vi "Begin.vi"(8 "error in":errorcluster) -> (0 "error out":errorcluster)   [LabVIEW 2016]
doc: "Called before other user functions, this VI is expected to open initial I/O refnums, load in file data, and do all program initialization. Notice that the <B>error out</B> terminal is simply used for data flow. Wiring it to other structures or subVIs ensures that this VI runs first."
uses:
  Refname/Queues.ctl
  Refname/Sensors.ctl
  Refname/Refname to String (Queues).vi
  Robot Global Data.vi
  Refname/Refname to String (Sensors).vi
  <vilib>/Rock Robotics/WPI/Joystick/WPI_JoystickDeviceEnum.ctl
  <vilib>/Rock Robotics/WPI/DriverStation/WPI_DriverStationRobotMode2.ctl
  <vilib>/Rock Robotics/WPI/ThirdParty/CanMotor/TalonSRX/WPI_CANTalonSRX_APIControlMode.ctl
  Refname/Motors.ctl
  <vilib>/Rock Robotics/WPI/SafetyOutput/WPI_SafetyOutputConfigMenu.ctl
  Refname/Controllers.ctl
  Refname/Refname to String (Motors).vi
  <vilib>/Rock Robotics/WPI/ThirdParty/CanMotor/TalonSRX/WPI_CANTalonSRX_APIFeedbackSelect.ctl
  <vilib>/Rock Robotics/WPI/ThirdParty/Sensors/ADIS16448 IMU/ADIS16448_IMU.lvlib
  <vilib>/Rock Robotics/SystemInterfaces/spilib/spi_bus.ctl
  Refname/Refname to String (Controllers).vi
panel:
  in  "Values to Log":string="TimeStamp, X, Y, Z, a, b, c, d, setpoint 1, setpoint 2, setpoint 3, setpoint 4, wheel power 1, wheel power 2, wheel power 3, wheel power 4, swerve current 1, swerve current 2, swerve current 3, swerve current 4"
  in  "PID gains":T1={"proportional gain (Kc)"=5.0, "integral time (Ti, min)"=0.032, "derivative time (Td, min)"=0.0} {"derivative time (Td, min)" format="%.3f"; "integral time (Ti, min)" format="%.8f"; "proportional gain (Kc)" format="%.8f"}
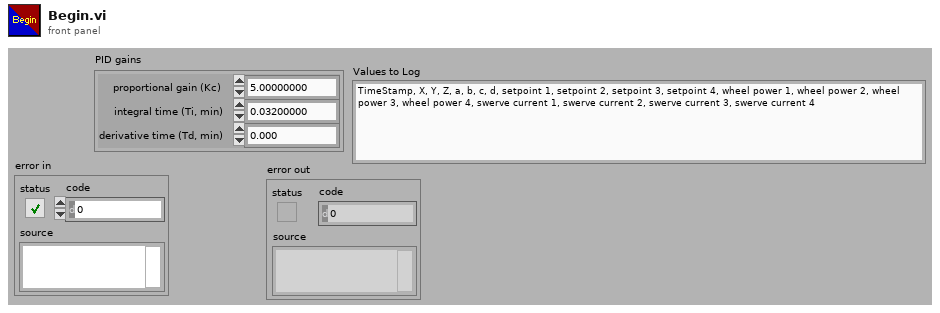
[diagram p1: front panel]
types:
  T1 = cluster{"proportional gain (Kc)":dbl, "integral time (Ti, min)":dbl, "derivative time (Td, min)":dbl}
  T2 = typedef "Queues.ctl" = enum16{"Log Queue"}
  T3 = cluster{"connection ID":refnum<k5>, "Running?":bool, "TCP Port":u16, "LastMessageReceivedTime":dbl, "WantsAppRestart":bool, "IsConnect":bool, "Vision Updates":cluster{"CapturedAgoMs":i32, "Valid?":bool, "CapturedAtTimestamp":dbl, "Targets":cluster{"X":dbl, "Y":dbl, "Z":dbl}[]}[]}
  T4 = typedef "WPI_SafetyOutputConfigMenu.ctl" = enum16{"Enable", "Disable"}
  T5 = typedef "Motors.ctl" = enum16{"Wheel 1", "Swerve 1", "Wheel 2", "Swerve 2", "Wheel 3", "Swerve 3", "Wheel 4", "Swerve 4", "Climber"}
  T6 = typedef "WPI_CANTalonSRX_APIControlMode.ctl" = enum8{"Percent VBus", "Speed", "Position", "Slave", "Unchanged / Invalid", "Voltage Compensation", "Current", "Motion Profile", "Motion Magic"}
  T7 = typedef "Sensors.ctl" = enum16{"DIP 1", "DIP 2", "DIP 3", "DIP 4", "IMU", "HuskieBoard"}
  T8 = typedef "spi_bus.ctl" = enum16{"SPI On-Board, CS0", "SPI On-Board, CS1", "SPI On-Board, CS2", "SPI On-Board, CS3", "SPI MXP", "Invalid"}
  T9 = typedef "WPI_DriverStationRobotMode2.ctl" = enum16{"Autonomous Disabled", "Autonomous Enabled", "Teleop Disabled", "Teleop Enabled", "Disconnected", "Finish", "Test Disabled", "Test Enabled", "Emergency Stopped"}
  T10 = typedef "WPI_CANTalonSRX_APIFeedbackSelect.ctl" = enum16{"Digital Quadrature Encoder", "Analog Potentiometer", "Analog Encoder", "Count on Quad-A (Rising-Edge)", "Count on Quad-A (Falling-Edge)", "CTR Magnetic Enc (Absolute)", "CTR Magnetic Enc (Relative)", "Pulse Width"}
  T11 = typedef "WPI_JoystickDeviceEnum.ctl" = enum16{"USB 0", "USB 1", "USB 2", "USB 3", "USB 4", "USB 5"}
  T12 = typedef "Controllers.ctl" = enum16{"Controller 0", "Controller 1"}
  T13 = typedef "WPI_MotorControlDeviceRef.ctl" = cluster{"DeviceStatus":errorcluster, "Type":T14, "PWM":cluster{"PWM Channel":T15, "DeadBand":T16}, "CAN":cluster{"Device Number":u8, "SetOutput VI Ref":variant, "GetOutput VI Ref":variant, "Enable VI Ref":variant, "Disable VI Ref":variant, "Data":variant}, "Invert":bool}
  T14 = typedef "WPI_MotorControlType.ctl" = enum16{"PWM", "CAN"}
  T15 = typedef "FPGA_DIOPWMChannel.ctl" = enum8{"PWM 0", "PWM 1", "PWM 2", "PWM 3", "PWM 4", "PWM 5", "PWM 6", "PWM 7", "PWM 8", "PWM 9", "PWM MXP 0", "PWM MXP 1", "PWM MXP 2", "PWM MXP 3", "PWM MXP 4", "PWM MXP 5", "PWM MXP 6", "PWM MXP 7", "PWM MXP 8", "PWM MXP 9", "Invalid"}
  T16 = typedef "WPI_PWMDeadband.ctl" = cluster{"Name":string, "maxPositivePwm":i32, "minPositivePwm":i32, "centerPwm":i32, "maxNegativePwm":i32, "minNegativePwm":i32, "angularRange":u16}
  T17 = typedef "WPI_JoystickDevRef.ctl" = cluster{"Device":T11}
  T18 = typedef "ADIS16448_IMU.lvlib/ADI_IMU_ADIS16448_InterruptDevRef.ctl" = cluster{"ADI IMU DevRef":T19, "InterruptRef":T20}
  T19 = typedef "ADIS16448_IMU.lvlib/ADI_IMU_ADIS16448_IMUDevRef.ctl" = cluster{"DevStatus":errorcluster, "Handle":i32, "SPI Bus":T8, "Device Found":bool, "Device Ready":bool, "Yaw Axis":enum16{"X", "Y", "Z"}, "AHRS Algorithm":enum16{"Complementary", "Madgwick"}, "Serial":u16, "Lot ID 2":u16, "Lot ID 1":u16, "Product ID":u16}
  T20 = typedef "WPI_InterruptRef.ctl" = cluster{"DevStatus":errorcluster, "InterruptIndex":T21}
  T21 = typedef "FPGA_InterruptIndex.ctl" = enum8{"0", "1", "2", "3", "4", "5", "6", "7", "Invalid"}
  T22 = typedef "WPI_SerialPortRef.ctl" = cluster{"DevStatus":errorcluster, "Serial Port Name":refnum<visa-resource-name>}
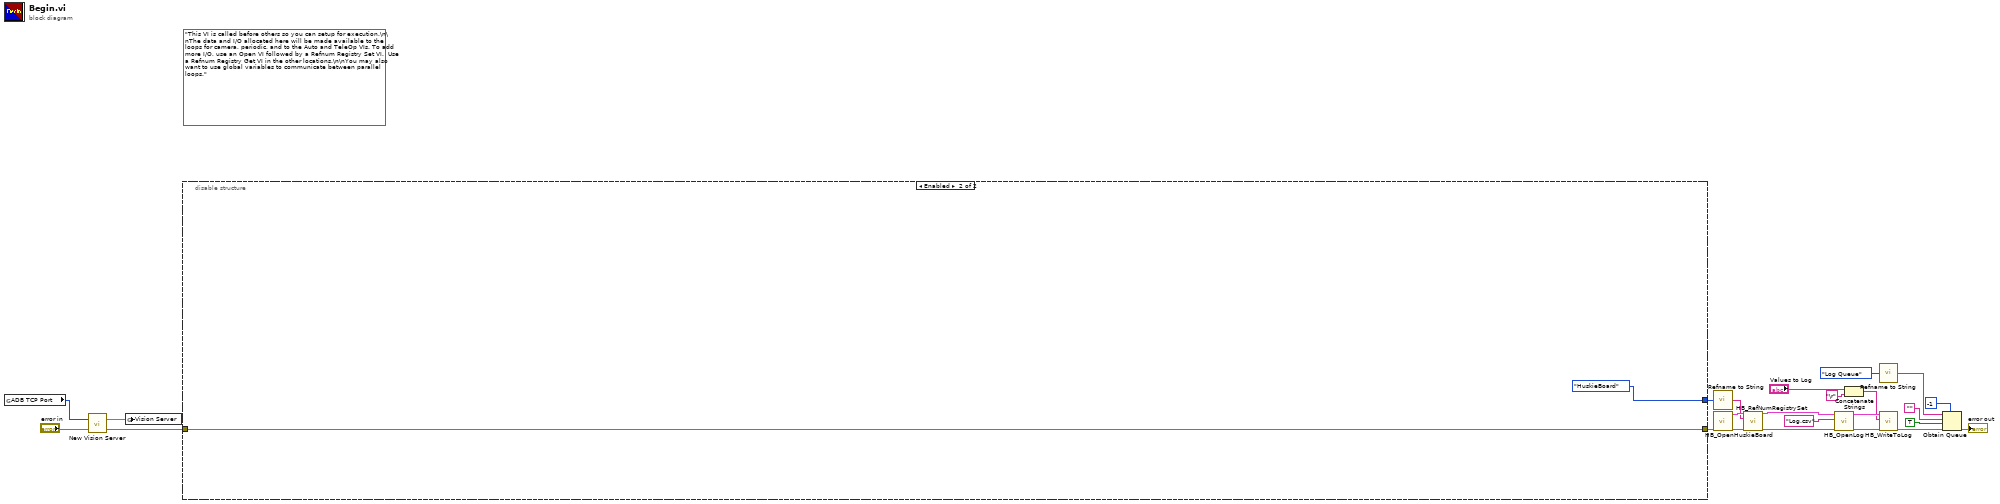
[diagram p0: block diagram]
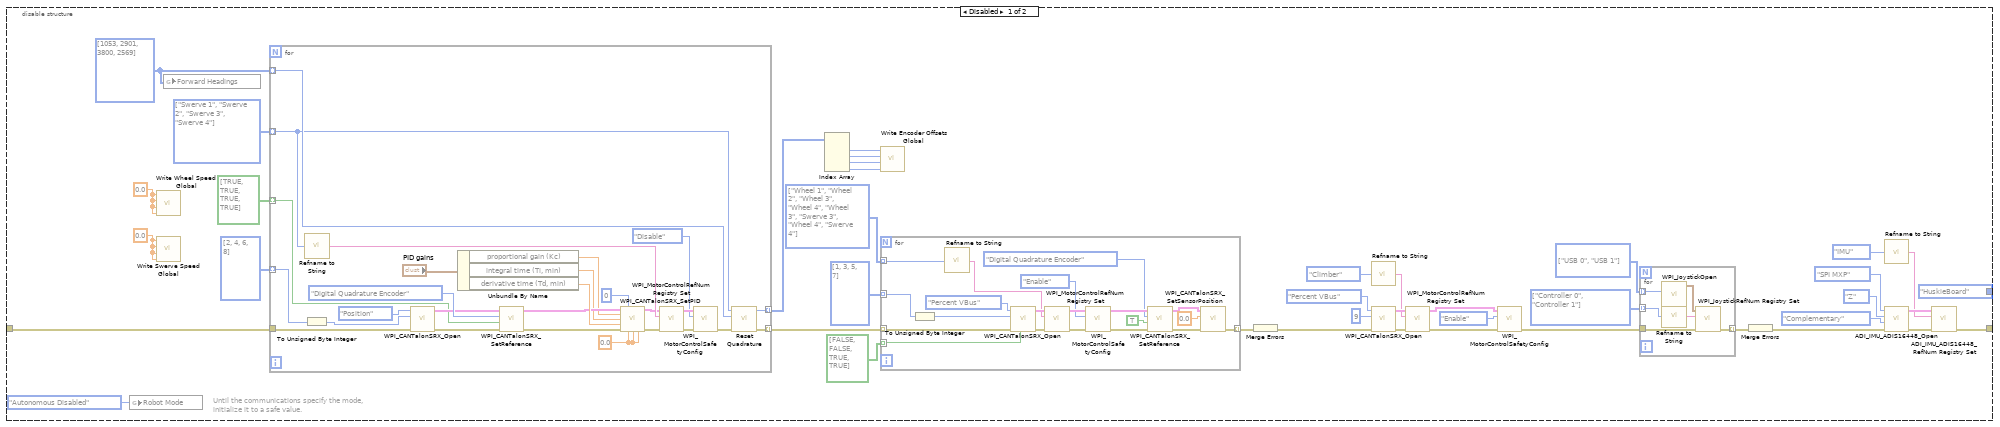
[diagram p2: hidden frame]
diagram:
  (unwired) "This VI is called before others so you can setup for execution.\n\nThe data and I/O allocated here will be made available to the loops for camera, periodic, and to the Auto and TeleOp VIs. To add more I/O, use an Open VI followed by a Refnum Registry Set VI.  Use a Refnum Registry Get VI in the other locations.\n\nYou may also want to use global variables to communicate between parallel loops."
  n1 = global read "Robot Global Data.vi" "ADB TCP Port"() -> (w11:u16)
  n2 = call "New Vision Server.vi"("error in"="error in", "TCP Port"=w11) -> ("error out"=w14:errorcluster, "Vision Server"=w13:T3)
  n3 = global write "Robot Global Data.vi" "Vision Server"(w13) -> ()
  n4 = disable-structure shown="Enabled" {
    disable-tunnel: [Sensors."HuskieBoard" ("Enum") Sensors."HuskieBoard" ("Enum")] -> w20
    disable-tunnel: w14 -> [w47 w121]
    disable-tunnel: [w46 w121] -> w10
    frame Disabled {
      w53 = i32[] [1053, 2901, 3800, 2569]
      w57 = 0.0
      w54 = 0.0
      w61 = T5[] [enum."Swerve 1", enum."Swerve 2", enum."Swerve 3", enum."Swerve 4"] items=["Wheel 1", "Swerve 1", "Wheel 2", "Swerve 2", "Wheel 3", "Swerve 3", "Wheel 4", "Swerve 4", "Climber"]
      w63 = T11[] [enum."USB 0", enum."USB 1"] items=["USB 0", "USB 1", "USB 2", "USB 3", "USB 4", "USB 5"]
      w64 = T12[] [enum."Controller 0", enum."Controller 1"] items=["Controller 0", "Controller 1"]
      w65 = T5[] [enum."Wheel 1", enum."Wheel 2", enum."Wheel 3", enum."Wheel 4", enum."Wheel 3", enum."Swerve 3", enum."Wheel 4", enum."Swerve 4"] items=["Wheel 1", "Swerve 1", "Wheel 2", "Swerve 2", "Wheel 3", "Swerve 3", "Wheel 4", "Swerve 4", "Climber"]
      # "Until the communications specify the mode,\ninitialize it to a safe value."
      n5 = global write "Robot Global Data.vi" "Robot Mode"(WPI_DriverStationRobotMode2."Autonomous Disabled" ("Robot Mode")) -> ()
      n6 = call "Write Wheel Speed Global.vi"("Wheel 4"=w54, "Wheel 3"=w54, "Wheel 2"=w54, "Wheel 1"=w54) -> ()
      n7 = call "Write Swerve Speed Global.vi"("Swerve 4"=w57, "Swerve 3"=w57, "Swerve 2"=w57, "Swerve 1"=w57) -> ()
      n8 = global write "Robot Global Data.vi" "Forward Headings"(w53) -> ()
      n9 = for {
        tunnel: w61 -> [w85] mode=indexing
        tunnel: i32[] [2, 4, 6, 8] -> [w88] mode=indexing
        tunnel: w47 -> [w87]
        tunnel: w53 -> [w86] mode=indexing
        tunnel: [w83] -> w55 mode=indexing
        tunnel: [w82] -> w58 mode=indexing
        tunnel: bool[] [TRUE, TRUE, TRUE, TRUE] -> [w77] mode=indexing
        w74 = 0.0 ("Output")
        n10 = To Unsigned Byte Integer(number=w88) -> (unsigned 8bit integer=w89:u8)
        n11 = call-poly "Refname to String.vi"("Enum"=w85) -> ("String"=w78:string)
        n12 = call <vilib>:"WPI_CANTalonSRX_Open.vi"("error in"=w87, "Device Number"=w89, "Control Mode"=WPI_CANTalonSRX_APIControlMode."Position") -> ("error out"=w79:errorcluster, "CAN Talon SRX Ref"=w80:T13)  [unwired: 7 in]
        n13 = Unbundle By Name("PID gains") -> ("proportional gain (Kc)"=w69:dbl, "integral time (Ti, min)"=w70:dbl, "derivative time (Td, min)"=w75:dbl)
        n14 = call <vilib>:"WPI_CANTalonSRX_SetReference.vi"("error in (no error)"=w79, "Reverse Feedback Sensor"=w77, "Feedback Reference"=WPI_CANTalonSRX_APIFeedbackSelect."Digital Quadrature Encoder", "CAN Talon SRX Ref"=w80) -> ("error out"=w72:errorcluster, "CAN Talon SRX Ref"=w73:T13)  [unwired: 6 in]
        n15 = call <vilib>:"WPI_CANTalonSRX_SetPID.vi"("CAN Talon SRX Ref"=w73, "Parameter Slot"=u8 0, "P"=w69, "I"=w70, "D"=w75, "error in (no error)"=w72, "F"=w74, "I Zone"=w74, "Ramp Rate"=w74) -> ("CAN Talon SRX Ref"=w67:T13, "error out"=w71:errorcluster)  [unwired: 5 in]
        n16 = call <vilib>:"WPI_MotorControlRefNum Registry Set.vi"("error in (no error)"=w71, "refnum name"=w78, "MotorControlDevRef"=w67) -> ("error out"=w92:errorcluster, "MotorControlDevRef"=w91:T13)  [unwired: 7 in]
        n17 = call <vilib>:"WPI_MotorControlSafetyConfig.vi"("error in (no error)"=w92, "mode"=WPI_SafetyOutputConfigMenu."Disable", "MotorControlDevRef"=w91) -> ("error out"=w84:errorcluster)  [unwired: 7 in, 1 out]
        n18 = call "Reset Quadrature.vi"("error in"=w84, "Forward Position"=w86, "Enum"=w85) -> ("error out"=w83:errorcluster, "Encoder Offset"=w82:i32)  [unwired: 7 in]
      }
      n19 = Index Array(array=w58) -> (element #1=w52:i32, element #2=w51:i32, element #3=w50:i32, element #4=w49:i32)  [unwired: 4 in]
      n20 = call "Write Encoder Offsets Global.vi"("Swerve 4"=w49, "Swerve 3"=w50, "Swerve 2"=w51, "Swerve 1"=w52) -> ()
      n21 = for {
        tunnel: w65 -> [w117] mode=indexing
        tunnel: i32[] [1, 3, 5, 7] -> [w109] mode=indexing
        tunnel: [w108] -> w30 mode=indexing
        tunnel: bool[] [FALSE, FALSE, TRUE, TRUE] -> [w107] mode=indexing
        tunnel: w55 -> [w106] mode=indexing
        n22 = To Unsigned Byte Integer(number=w109) -> (unsigned 8bit integer=w111:u8)
        n23 = call-poly "Refname to String.vi"("Enum"=w117) -> ("String"=w116:string)
        n24 = call <vilib>:"WPI_CANTalonSRX_Open.vi"("Invert"=w107, "error in"=w106, "Device Number"=w111, "Control Mode"=WPI_CANTalonSRX_APIControlMode."Percent VBus") -> ("error out"=w112:errorcluster, "CAN Talon SRX Ref"=w118:T13)  [unwired: 6 in]
        n25 = call <vilib>:"WPI_MotorControlRefNum Registry Set.vi"("error in (no error)"=w112, "refnum name"=w116, "MotorControlDevRef"=w118) -> ("error out"=w115:errorcluster, "MotorControlDevRef"=w114:T13)  [unwired: 7 in]
        n26 = call <vilib>:"WPI_MotorControlSafetyConfig.vi"("error in (no error)"=w115, "mode"=WPI_SafetyOutputConfigMenu."Enable", "MotorControlDevRef"=w114) -> ("error out"=w103:errorcluster, "MotorControlDevRef"=w102:T13)  [unwired: 7 in]
        n27 = call <vilib>:"WPI_CANTalonSRX_SetReference.vi"("error in (no error)"=w103, "Reverse Feedback Sensor"=TRUE, "Feedback Reference"=WPI_CANTalonSRX_APIFeedbackSelect."Digital Quadrature Encoder", "CAN Talon SRX Ref"=w102) -> ("error out"=w105:errorcluster, "CAN Talon SRX Ref"=w104:T13)  [unwired: 6 in]
        n28 = call <vilib>:"WPI_CANTalonSRX_SetSensorPosition.vi"("error in (no error)"=w105, "New Sensor Position"=0.0, "CAN Talon SRX Ref"=w104) -> ("error out"=w108:errorcluster)  [unwired: 7 in, 1 out]
      }
      n29 = Merge Errors(w30) -> (w31:errorcluster)
      n30 = call-poly "Refname to String.vi"("Enum"=Motors."Climber") -> ("String"=w27:string)
      n31 = call <vilib>:"WPI_CANTalonSRX_Open.vi"("error in"=w31, "Device Number"=u8 9, "Control Mode"=WPI_CANTalonSRX_APIControlMode."Percent VBus") -> ("error out"=w33:errorcluster, "CAN Talon SRX Ref"=w32:T13)  [unwired: 7 in]
      n32 = call <vilib>:"WPI_MotorControlRefNum Registry Set.vi"("error in (no error)"=w33, "refnum name"=w27, "MotorControlDevRef"=w32) -> ("error out"=w35:errorcluster, "MotorControlDevRef"=w34:T13)  [unwired: 7 in]
      n33 = call <vilib>:"WPI_MotorControlSafetyConfig.vi"("error in (no error)"=w35, "mode"=WPI_SafetyOutputConfigMenu."Enable", "MotorControlDevRef"=w34) -> ("error out"=w36:errorcluster)  [unwired: 7 in, 1 out]
      n34 = for {
        tunnel: w64 -> [w99] mode=indexing
        tunnel: w63 -> [w97] mode=indexing
        tunnel: [w95] -> w42 mode=indexing
        tunnel: w36 -> [w94]
        n35 = call <vilib>:"WPI_JoystickOpen.vi"("JoystickDevice"=w97) -> ("JoystickDevRef"=w96:T17)  [unwired: 10 in]
        n36 = call-poly "Refname to String.vi"("Enum"=w99) -> ("string"=w98:string)
        n37 = call <vilib>:"WPI_JoystickRefNum Registry Set.vi"("error in (no error)"=w94, "refnum name"=w98, "JoystickDevRef"=w96) -> ("error out"=w95:errorcluster)  [unwired: 7 in, 1 out]
      }
      n38 = Merge Errors(w42) -> (w43:errorcluster)
      n39 = call-poly "Refname to String.vi"("Enum"=Sensors."IMU") -> ("String"=w38:string)
      n40 = call <vilib>:"ADI_IMU_ADIS16448_Open.vi"("error in"=w43, "AHRS Algorithm"=enum16{"Complementary", "Madgwick"}."Complementary", "Yaw Axis"=enum16{"X", "Y", "Z"}."Z", "SPI Chip Select"=spi_bus."SPI MXP") -> ("error out"=w45:errorcluster, "ADI IMU Interrupt DevRef"=w44:T18)  [unwired: 6 in]
      n41 = call <vilib>:"ADI_IMU_ADIS16448_RefNum Registry Set.vi"("error in (no error)"=w45, "refnum name"=w38, "ADI IMU Interrupt DevRef"=w44) -> ("error out"=w46:errorcluster)  [unwired: 7 in, 1 out]
    }
    frame Enabled {
    }
  }
  n42 = call-poly "Refname to String.vi"("Enum"=w20) -> ("String"=w21:string)
  n43 = call <vilib>:"HB_OpenHuskieBoard.vi"("error in (no error)"=w10) -> ("error out"=w23:errorcluster, "HBDeviceRef"=w22:T22)  [unwired: 9 in]
  n44 = call <vilib>:"HB_RefNumRegistrySet.vi"("HBDevRef"=w22, "refnum name"=w21, "error in (no error)"=w23) -> ("HBDevRef"=w7:T22, "error out"=w6:errorcluster)  [unwired: 11 in]
  n45 = call <vilib>:"HB_OpenLog.vi"("error in (no error)"=w6, "File Name"="Log.csv", "HBDeviceRef"=w7) -> ("error out"=w9:errorcluster, "HBDeviceRef"=w8:T22)  [unwired: 7 in]
  n46 = Concatenate Strings("Values to Log", "\r") -> (w3:string)
  n47 = call-poly "Refname to String.vi"("Enum"=Queues."Log Queue") -> ("String"=w19:string)
  n48 = call <vilib>:"HB_WriteToLog.vi"("error in (no error)"=w9, "Log string"=w3, "HBDevRef"=w8) -> ("error out"=w4:errorcluster)  [unwired: 7 in, 1 out]
  n49 = Obtain Queue(max queue size (-1, unlimited)=-1, name (unnamed)=w19, element data type="", create if not found? (T)=TRUE, error in (no error)=w4) -> (error out=→"error out":errorcluster)  [unwired: 2 out]
